vi "cvt_String_TagList.vi"(8 "error in (no error)":errorcluster, 9 "Tag Name":string, 10 "Tag List":T1[](array[typedef]), 11 "Method":T3=enum."getindex") -> (0 "error out":errorcluster, 1 "Index":i32, 2 "Default Data":string[](array[string]), 3 "Tag Description":string, 5 "String Tag List":T1[](array[typedef]))   [LabVIEW 2010]
uses:
  TypeDefs/cvt_TagList Methods.ctl
  TypeDefs/cvt_Tag Configuration.ctl
  TypeDefs/cvt_Data Types.ctl
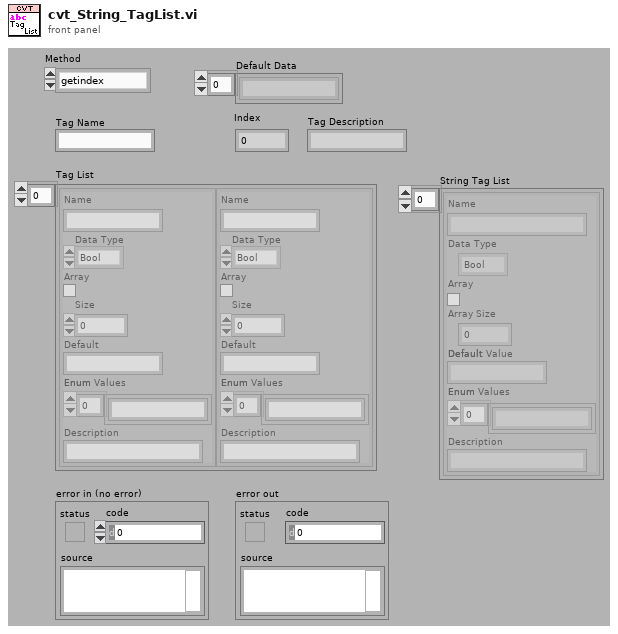
[diagram p1: front panel]
types:
  T1 = typedef "cvt_Tag Configuration.ctl" = cluster{"Name":string, "Data Type":T2, "Array":bool, "Size":u32, "Default":string, "Enum":string[], "Description":string}
  T2 = typedef "cvt_Data Types.ctl" = enum16{"Bool", "U8", "I32", "Double", "String", "Enum"}
  T3 = typedef "cvt_TagList Methods.ctl" = enum16{"init", "getindex", "getdesc", "getlist"}
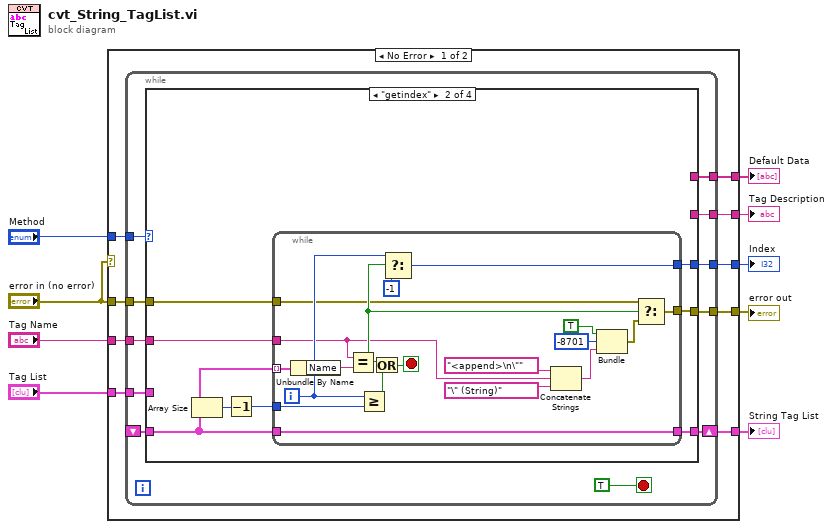
[diagram p0: block diagram]
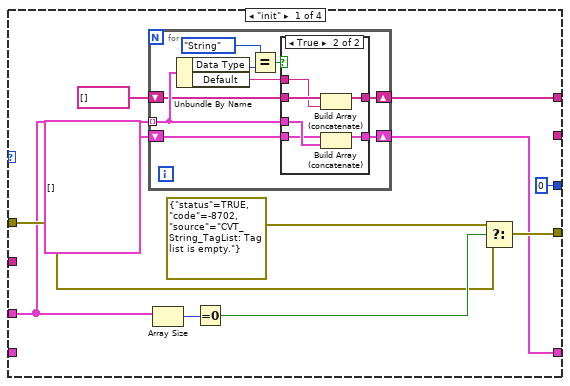
[diagram p2: hidden frame]
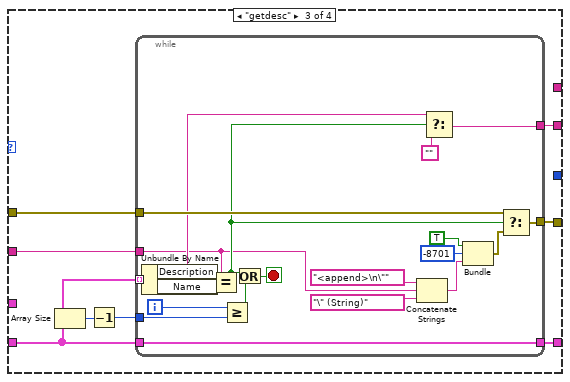
[diagram p4: hidden frame]
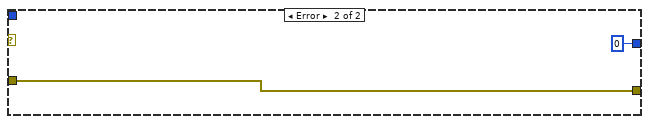
[diagram p6: hidden frame]
diagram:
  n1 = case shown="No Error" "error in (no error)" {
    tunnel: "Method" -> [w18 _]
    tunnel: "Tag Name" -> [w17 _]
    tunnel: [w16 w116] -> w7
    tunnel: "error in (no error)" -> [w15 w116]
    tunnel: "Tag List" -> [w14 _]
    tunnel: [w13 0 ("f")] -> w4
    tunnel: [w12 _] -> w3
    tunnel: [w11 _] -> w2
    tunnel: [w10 _] -> w1
    frame No Error {
      n2 = while {
        tunnel: w18 -> [w28]
        tunnel: w17 -> [w27]
        tunnel: w15 -> [w26]
        tunnel: [w25] -> w16
        tunnel: w14 -> [w22]
        shift-right: [w24] -> w10
        shift-left: _ -> [w23]
        tunnel: [w21] -> w13
        tunnel: [w20] -> w12
        tunnel: [w19] -> w11
        stop <- TRUE stop-if-true
        n3 = case shown="\"getindex\"" w28 {
          tunnel: w27 -> [_ w65 w92 _]
          tunnel: w26 -> [w37 w59 w86 w113]
          tunnel: [w39 w60 w87 w113] -> w25
          tunnel: [w33 w62 w89 w114] -> w24
          tunnel: w23 -> [_ w61 w88 w114]
          tunnel: w22 -> [w34 _ _ _]
          tunnel: [0 ("f") w58 _ _] -> w21
          tunnel: [w30 _ _ _] -> w20
          tunnel: [_ _ w85 _] -> w19
          frame "init" {
            n4 = for {
              tunnel: w34 -> [w45] mode=indexing
              shift-right: [w43] -> w33
              shift-left: T1[] [] -> [w44]
              shift-right: [w41] -> w30
              shift-left: string[] [] -> [w42]
              n5 = Unbundle By Name(w45) -> ("Data Type"=w49:T2, "Default"=w46:string)
              n6 = Equal?(x=cvt_Data_Types."String", y=w49) -> (x = y?=w48:bool)
              n7 = case shown="True" w48 {
                tunnel: w46 -> [_ w52]
                tunnel: w42 -> [w50 w57]
                tunnel: [w50 w56] -> w41
                tunnel: w45 -> [_ w55]
                tunnel: w44 -> [w51 w54]
                tunnel: [w51 w53] -> w43
                frame False {
                }
                frame True {
                  n8 = Build Array (concatenate)(w57, w52) -> (w56:string[])
                  n9 = Build Array (concatenate)(w54, w55) -> (w53:T1[])
                }
              }
            }
            n10 = Array Size(array=w34) -> (size(s)=w40:i32)
            n11 = Equal To 0?(x=w40) -> (x = 0?=w38:bool)
            n12 = Select(t=errorcluster {"status"=TRUE, "code"=-8702, "source"="CVT_String_TagList: Tag list is empty."} ("f"), s=w38, f=w37) -> (s? t:f=w39:errorcluster)
          }
          frame "getindex" {
            n13 = Array Size(array=w61) -> (size(s)=w64:i32)
            n14 = Decrement(x=w64) -> (x-1=w63:i32)
            n15 = while {
              tunnel: w61 -> [w84] mode=indexing
              tunnel: w65 -> [w66]
              tunnel: w63 -> [w82]
              tunnel: [w73] -> w58
              tunnel: [w76] -> w62
              tunnel: w61 -> [w76]
              tunnel: [w75] -> w60
              tunnel: w59 -> [w74]
              i -> [w79]
              stop <- w80 stop-if-true
              n16 = Unbundle By Name(w84) -> ("Name"=w83:string)
              n17 = Equal?(x=w66, y=w83) -> (x = y?=w77:bool)
              n18 = Greater Or Equal?(x=w79, y=w82) -> (x >= y?=w81:bool)
              n19 = Or(x=w77, y=w81) -> (x .or. y?=w80:bool)
              n20 = Select(t=w79, s=w77, f=-1) -> (s? t:f=w73:i32)
              n21 = Concatenate Strings("<append>\n\"" ("source"), w66, "\" (String)" ("source")) -> (w71:string)
              n22 = Bundle("status"=TRUE, "code"=-8701, w71) -> (w67:cluster{"status":bool, "code":i32, string})  [unwired: 1 out]
              n23 = Select(t=w74, s=w77, f=w67) -> (s? t:f=w75:errorcluster)
            }
          }
          frame "getdesc" {
            n24 = Array Size(array=w88) -> (size(s)=w91:i32)
            n25 = Decrement(x=w91) -> (x-1=w90:i32)
            n26 = while {
              tunnel: w88 -> [w112] mode=indexing
              tunnel: w92 -> [w93]
              tunnel: w90 -> [w110]
              tunnel: [w106] -> w89
              tunnel: w88 -> [w106]
              tunnel: [w105] -> w87
              tunnel: w86 -> [w104]
              tunnel: [w102] -> w85
              i -> [w107]
              stop <- w108 stop-if-true
              n27 = Unbundle By Name(w112) -> ("Description"=w101:string, "Name"=w111:string)
              n28 = Equal?(x=w93, y=w111) -> (x = y?=w100:bool)
              n29 = Greater Or Equal?(x=w107, y=w110) -> (x >= y?=w109:bool)
              n30 = Or(x=w100, y=w109) -> (x .or. y?=w108:bool)
              n31 = Concatenate Strings("<append>\n\"" ("source"), w93, "\" (String)" ("source")) -> (w96:string)
              n32 = Select(t=w101, s=w100, f="") -> (s? t:f=w102:string)
              n33 = Bundle("status"=TRUE, "code"=-8701, w96) -> (w94:cluster{"status":bool, "code":i32, string})  [unwired: 1 out]
              n34 = Select(t=w104, s=w100, f=w94) -> (s? t:f=w105:errorcluster)
            }
          }
          frame "getlist" {
          }
        }
      }
    }
    frame Error {
    }
  }
  "error out" <- w7
  "Index" <- w4
  "Default Data" <- w3
  "Tag Description" <- w2
  "String Tag List" <- w1
